vi "Relative Error calc.vi"(1 "X":dbl, 2 "Xk":dbl, 3 "d":dbl, 4 "c":dbl) -> (0 "Относительная погрешность, %":dbl)   [LabVIEW 2013]
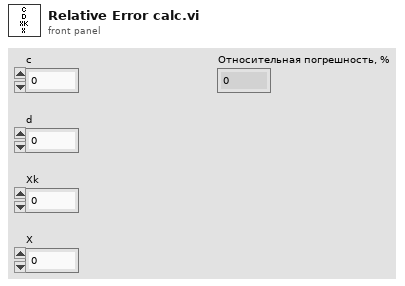
[diagram p1: front panel]
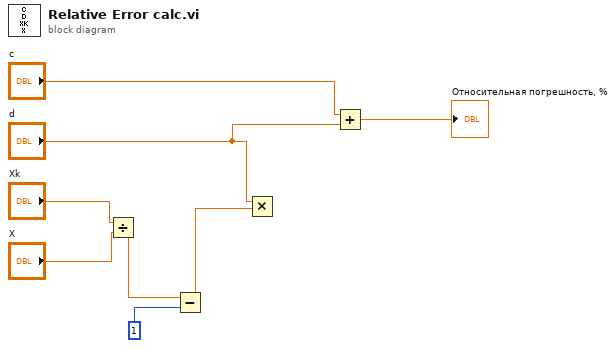
[diagram p0: block diagram]
diagram:
  n1 = Divide(x="Xk", y="X") -> (x/y=w6:dbl)
  n2 = Subtract(x=w6, y=1) -> (x-y=w4:dbl)
  n3 = Multiply(x="d", y=w4) -> ()  [unwired: 1 out]
  n4 = Add(x="c", y="d") -> (x+y=→"Относительная погрешность, %":dbl)
